vi "read.vi"() -> ()   [LabVIEW 2014]
uses:
  <vilib>/Instr/_visa.llb/VISA Configure Serial Port (Instr).vi
panel:
  in  "VISA resource name 2":refnum<visa-resource-name>
  out "Threshold sent":bool
  out "Pass Ack 3":bool
  out "Pass Ack 2":bool
  out "Pass Ack":bool
  out "password is wrong":bool
  in  "Tab Control 2":enum32{"Page 1", "Page 2", "Page 3"}(tab)
  in  "Password":string
  in  "Threshold":string
  out "read buffer":string
  out "Iteration":i32
  out "return count read":u32
  out "PC on Ack":bool
  in  "Reset":bool
  out "Reset#":i32
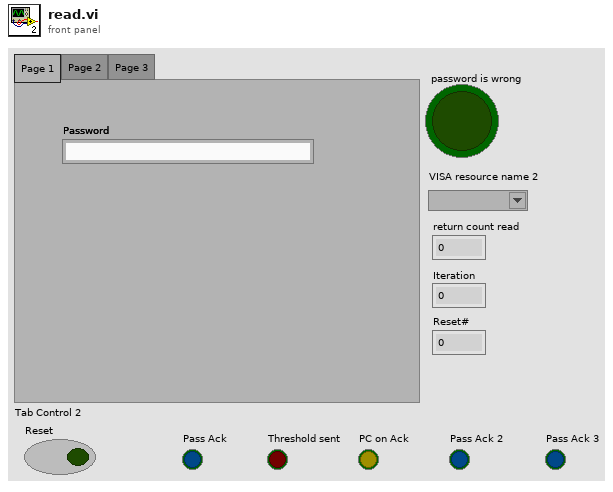
[diagram p1: front panel]
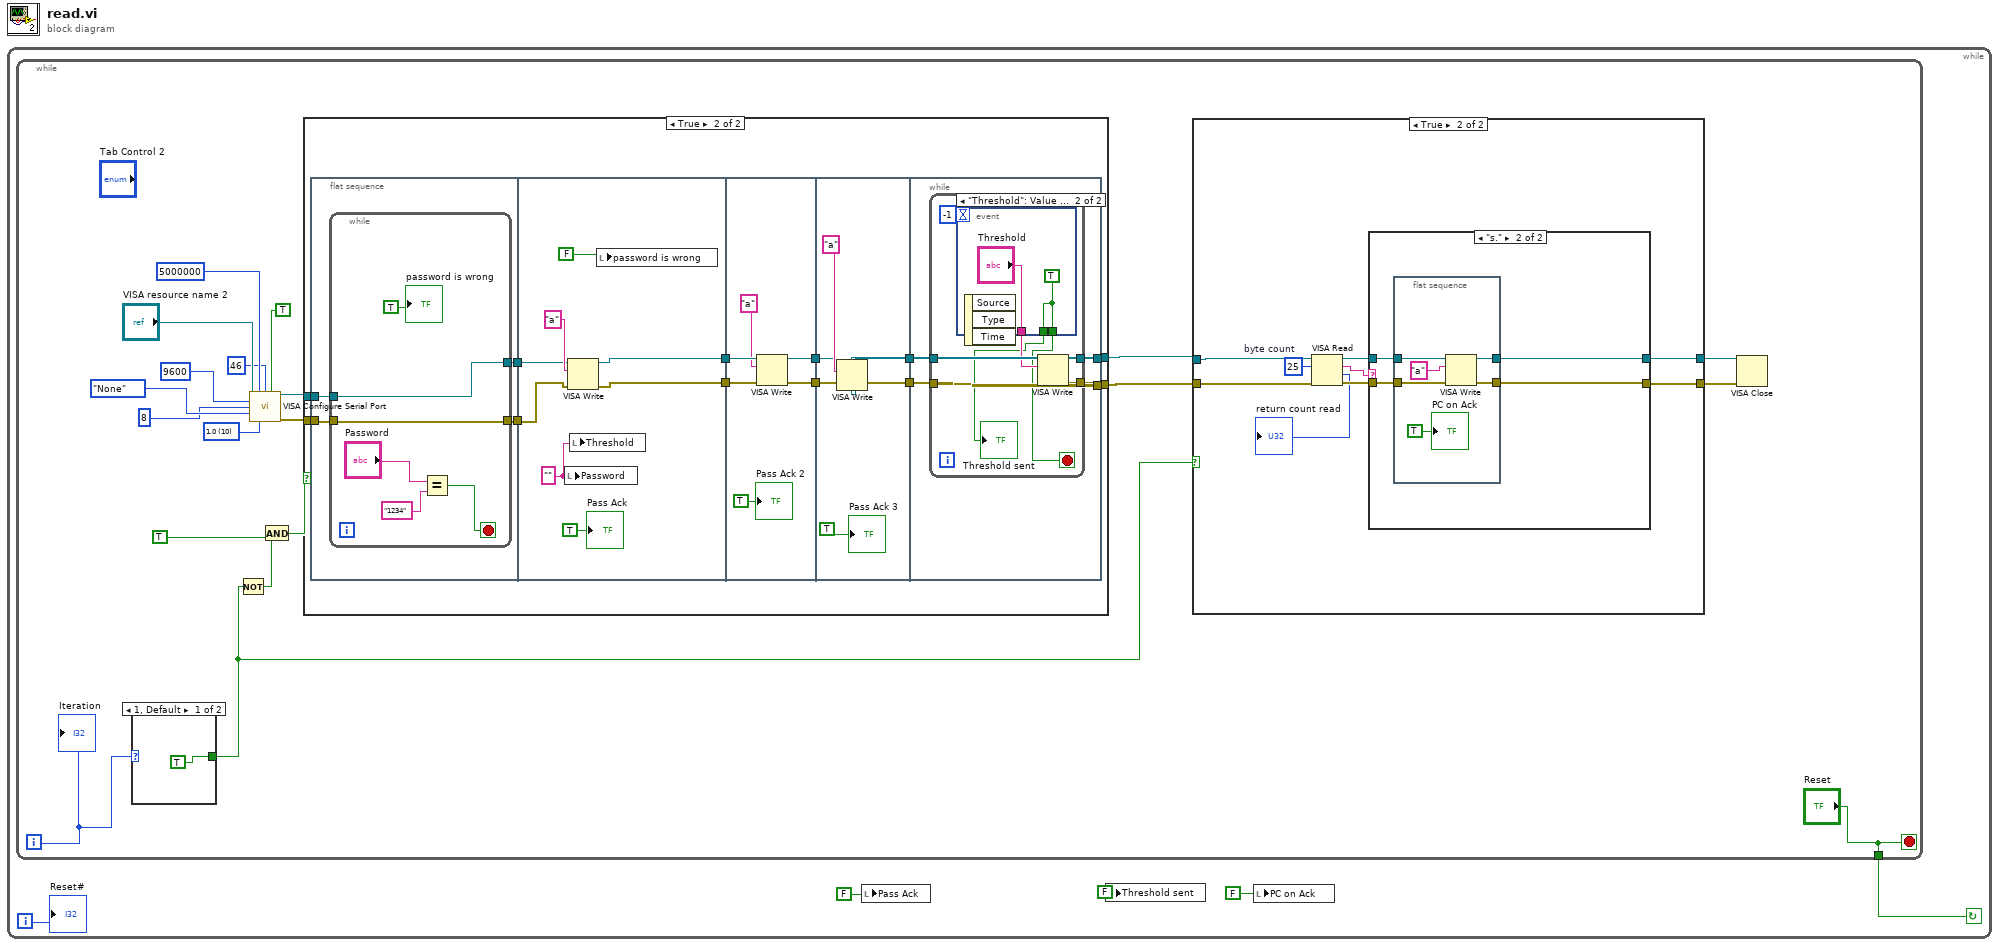
[diagram p0: block diagram]
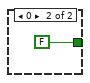
[diagram p2: hidden frame]
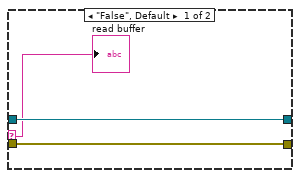
[diagram p4: hidden frame]
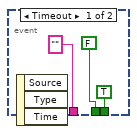
[diagram p6: hidden frame]
diagram:
  n1 = while {
    i -> [w5]
    stop <- w4 continue-if-true
    n2 = while {
      tunnel: ["Reset"] -> w4
      i -> [w9]
      stop <- "Reset" stop-if-true
      w22 = u16 10 items=["1.0"=10, "1.5"=15, "2.0"=20] ("stop bits (10: 1 bit)")
      n3 = case shown="1, Default" w9 {
        tunnel: [TRUE FALSE] -> w8
        frame 1, Default {
        }
        frame 0 {
        }
      }
      n4 = Not(x=w8) -> (.not. x?=w17:bool)
      n5 = call-poly "VISA Configure Serial Port"("VISA resource name"="VISA resource name 2", "timeout (10sec)"=u32 5000000, "termination char\n(0xA = '\\n' = LF)"=u8 46 ("termination char\n(0xA = '\\n' = LF)"), "Enable Termination\nChar (T)"=TRUE ("Enable Termination\nChar (T)"), "baud rate (9600)"=u32 9600, "data bits (8)"=u16 8, "parity (0:none)"=enum16{"None", "Odd", "Even", "Mark", "Space"}."None", "stop bits (10: 1 bit)"=w22) -> ("VISA resource name out"=w16:refnum<visa-resource-name>, "error out"=w15:errorcluster)  [unwired: 6 in]
      n6 = And(x=w17, y=TRUE) -> (x .and. y?=w14:bool)
      n7 = case shown="True" w14 {
        tunnel: w15 -> [w53 w65]
        tunnel: [w52 w63] -> w13
        tunnel: [w53 w62] -> w11
        tunnel: w16 -> [w52 w64]
        frame False {
        }
        frame True {
          n8 = flat-sequence {
            tunnel: w65 -> [w69]
            tunnel: w64 -> [w68]
            tunnel: [w67] -> w61
            tunnel: [w66] -> w60
            tunnel: w61 -> [w83]
            tunnel: w60 -> [w76]
            tunnel: [w82] -> w59
            tunnel: [w81] -> w58
            tunnel: w59 -> [w86]
            tunnel: w58 -> [w89]
            tunnel: [w88] -> w57
            tunnel: [w87] -> w55
            tunnel: w57 -> [w91]
            tunnel: [w94] -> w56
            tunnel: w55 -> [w92]
            tunnel: [w93] -> w54
            tunnel: [w98] -> w63
            tunnel: [w97] -> w62
            tunnel: w56 -> [w99]
            tunnel: w54 -> [w96]
            frame #0 {
              n9 = while {
                tunnel: w69 -> [w73]
                tunnel: w68 -> [w72]
                tunnel: [w73] -> w67
                tunnel: [w72] -> w66
                stop <- w74 stop-if-true
                n10 = Equal?(x="Password", y="1234") -> (x = y?=w74:bool)
                "password is wrong" <- TRUE
              }
            }
            frame #1 {
              w78 = "" ("Password")
              n11 = local write "Password"(w78) -> ()
              n12 = VISA Write(VISA resource name=w76, write buffer="a", error in (no error)=w83) -> (VISA resource name out=w82:refnum<visa-resource-name>, error out=w81:errorcluster)  [unwired: 1 out]
              n13 = local write "Threshold"(w78) -> ()
              n14 = local write "password is wrong"(FALSE) -> ()
              "Pass Ack" <- TRUE ("Pass Ack")
            }
            frame #2 {
              n15 = VISA Write(VISA resource name=w86, write buffer="a", error in (no error)=w89) -> (VISA resource name out=w88:refnum<visa-resource-name>, error out=w87:errorcluster)  [unwired: 1 out]
              "Pass Ack 2" <- TRUE ("Pass Ack")
            }
            frame #3 {
              n16 = VISA Write(VISA resource name=w91, write buffer="a", error in (no error)=w92) -> (VISA resource name out=w94:refnum<visa-resource-name>, error out=w93:errorcluster)  [unwired: 1 out]
              "Pass Ack 3" <- TRUE ("Pass Ack")
            }
            frame #4 {
              n17 = while {
                tunnel: w99 -> [w107]
                tunnel: [w106] -> w98
                tunnel: [w105] -> w97
                tunnel: w96 -> [w100]
                stop <- w102 stop-if-true
                n18 = event shown="[1] \"Threshold\": Value Change" {
                  selector: _ -> [_ _]
                  dyn-events: _ -> [_ _]
                  timeout: -1 -> [_ _]
                  tunnel: [TRUE w111] -> w102
                  tunnel: ["" "Threshold"] -> w104
                  tunnel: [FALSE w111] -> w101
                  event Timeout {
                    n19 = event-data() -> ()  [unwired: 1 in, 3 out]
                  }
                  event "Threshold": Value Change {
                    w111 = TRUE
                    n20 = event-data() -> ()  [unwired: 1 in, 3 out]
                  }
                }
                "Threshold sent" <- w101
                n21 = VISA Write(VISA resource name=w107, write buffer=w104, error in (no error)=w100) -> (VISA resource name out=w106:refnum<visa-resource-name>, error out=w105:errorcluster)  [unwired: 1 out]
              }
            }
          }
        }
      }
      n22 = case shown="True" w8 {
        tunnel: [w29 w36] -> w12
        tunnel: [w28 w38] -> w10
        tunnel: w13 -> [w29 w37]
        tunnel: w11 -> [w28 w33]
        frame False {
        }
        frame True {
          w31 = u32 25  # byte count
          n23 = VISA Read(VISA resource name=w37, byte count=w31, error in (no error)=w33) -> (VISA resource name out=w34:refnum<visa-resource-name>, read buffer=w30:string, return count=→"return count read":u32, error out=w35:errorcluster)
          n24 = case shown="\"s.\"" w30 {
            selector: w30 -> [w39 _]
            tunnel: [w40 w42] -> w38
            tunnel: [w41 w43] -> w36
            tunnel: w35 -> [w40 w44]
            tunnel: w34 -> [w41 w45]
            frame "False", Default {
              "read buffer" <- w39
            }
            frame "s." {
              n25 = flat-sequence {
                tunnel: [w48] -> w43
                tunnel: [w47] -> w42
                tunnel: w45 -> [w50]
                tunnel: w44 -> [w49]
                frame #0 {
                  n26 = VISA Write(VISA resource name=w50, write buffer="a", error in (no error)=w49) -> (VISA resource name out=w48:refnum<visa-resource-name>, error out=w47:errorcluster)  [unwired: 1 out]
                  "PC on Ack" <- TRUE ("PC on Ack")
                }
              }
            }
          }
        }
      }
      n27 = VISA Close(VISA resource name=w12, error in (no error)=w10) -> ()  [unwired: 1 out]
      "Iteration" <- w9
    }
    n28 = local write "Pass Ack"(FALSE) -> ()
    n29 = local write "Threshold sent"(FALSE ("Pass Ack")) -> ()
    n30 = local write "PC on Ack"(FALSE) -> ()
    "Reset#" <- w5
  }
